vi "Agilent 2000 3000 X-Series Edge Triggered Acquisition.vi"() -> ()   [LabVIEW 2015]
doc: "This example shows how to configure the oscilloscope to perform an edge-triggered waveform acquisition."
uses:
  Agilent 2000 3000 X-Series.lvlib
panel:
  in  "Channel Name (0: Channel 1)":i32(ring) items=["Channel 1", "Channel 2", "Channel 3", "Channel 4"]
  in  "Coupling (1: DC)":i32(ring)=1 items=["AC", "DC"]
  in  "Time per Division (0.0005 s)":dbl=0.0005
  in  "Probe Attenuation (1.0)":dbl=10.0
  in  "Vertical Range (1.0 V)":dbl=1.0
  in  "Trigger Level (0.0 V)":dbl
  out "Waveform Data":waveform(dbl)(graph)
  in  "VISA resource name":refnum<visa-resource-name>
  # "(c) 2011-2023 National Instruments.  ALL RIGHTS RESERVED."
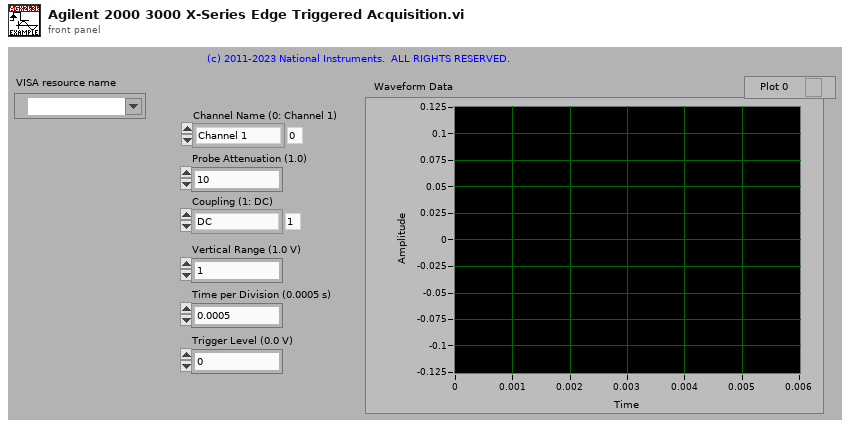
[diagram p1: front panel]
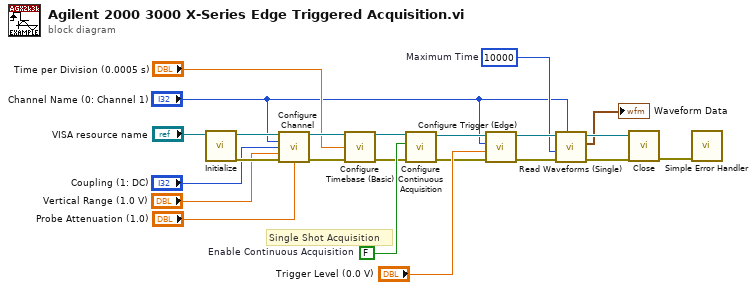
[diagram p0: block diagram]
diagram:
  w2 = u32 10000  # Maximum Time
  w12 = FALSE  # Enable Continuous Acquisition
  # "Single Shot Acquisition"
  n1 = call "Initialize.vi"("VISA resource name"="VISA resource name") -> ("error out"=w20:errorcluster, "VISA resource name out"=w21:refnum<visa-resource-name>)  [unwired: 4 in, 5 out]
  n2 = call "Configure Channel.vi"("VISA resource name"=w21, "Channel Name (0: Channel 1)"="Channel Name (0: Channel 1)", "Coupling (1: DC)"="Coupling (1: DC)", "Vertical Range (40.0 V)"="Vertical Range (1.0 V)", "error in (no error)"=w20, "Probe Attenuation (1.0)"="Probe Attenuation (1.0)") -> ("VISA resource name out"=w15:refnum<visa-resource-name>, "error out"=w16:errorcluster)  [unwired: 5 in, 3 out]
  n3 = call "Configure Timebase (Basic).vi"("VISA resource name"=w15, "Scale (50 s/div)"="Time per Division (0.0005 s)", "error in (no error)"=w16) -> ("VISA resource name out"=w13:refnum<visa-resource-name>, "error out"=w11:errorcluster)  [unwired: 6 in, 5 out]
  n4 = call "Configure Continuous Acquisition.vi"("error in (no error)"=w11, "Enable Continuous Acquisition Mode (T:Enable)"=w12, "VISA resource name"=w13) -> ("error out"=w5:errorcluster, "VISA resource name out"=w6:refnum<visa-resource-name>)  [unwired: 7 out]
  n5 = call "Configure Trigger (Edge).vi"("error in (no error)"=w5, "Trigger Level (0 V)"="Trigger Level (0.0 V)", "Trigger Source (0: Channel 1)"="Channel Name (0: Channel 1)", "VISA resource name"=w6) -> ("error out"=w8:errorcluster, "VISA resource name out"=w4:refnum<visa-resource-name>)  [unwired: 3 in, 3 out]
  n6 = call "Read Waveforms (Single).vi"("Bind Source Channel (2: None)"="Channel Name (0: Channel 1)", "error in (no error)"=w8, "Timeout (10000 ms)"=w2, "VISA resource name"=w4) -> ("error out"=w9:errorcluster, "Waveform Data"=→"Waveform Data":waveform(dbl), "VISA resource name out"=w10:refnum<visa-resource-name>)  [unwired: 1 in, 4 out]
  n7 = call "Close.vi"("error in (no error)"=w9, "VISA resource name"=w10) -> ("error out"=w23:errorcluster)  [unwired: 9 out]
  n8 = call <vilib>:"Simple Error Handler.vi"("error in (no error)"=w23) -> ()  [unwired: 1 in, 8 out]
